vi "MonoSpec50 Find Ref Position_trig.vi"(2 "error in":errorcluster, 4 "Moving Ref":refnum<vi>) -> (0 "error out":errorcluster, 1 "Moving":bool caption="Déplacement\nen cours")   [LabVIEW 2012]
doc: "Ce VI envoie un train d'impulsion au moteur, pour le faire tourné dans la direction négative. Les impulsion sont générée en continu jusqu'à ce qu'un front montant soit détecté sur la ligne de détection de position de référence."
uses:
  <vilib>/Utility/error.llb/DialogType.ctl
  <vilib>/DAQmx/write.llb/DAQmx Write (Digital Bool 1Line 1Point).vi
  <vilib>/DAQmx/read.llb/DAQmx Read (Counter U32 1Chan 1Samp).vi
  <vilib>/DAQmx/miscellaneous.llb/DAQmx Fill In Error Info.vi
  <resource>/objmgr/daqmx.rc
panel:
  out "End":bool=TRUE
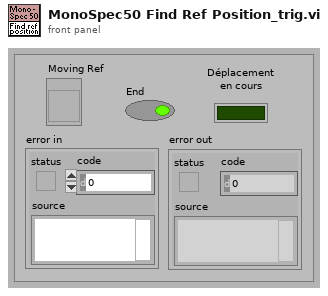
[diagram p1: front panel]
types:
  T1 = typedef "DialogType.ctl" = u16
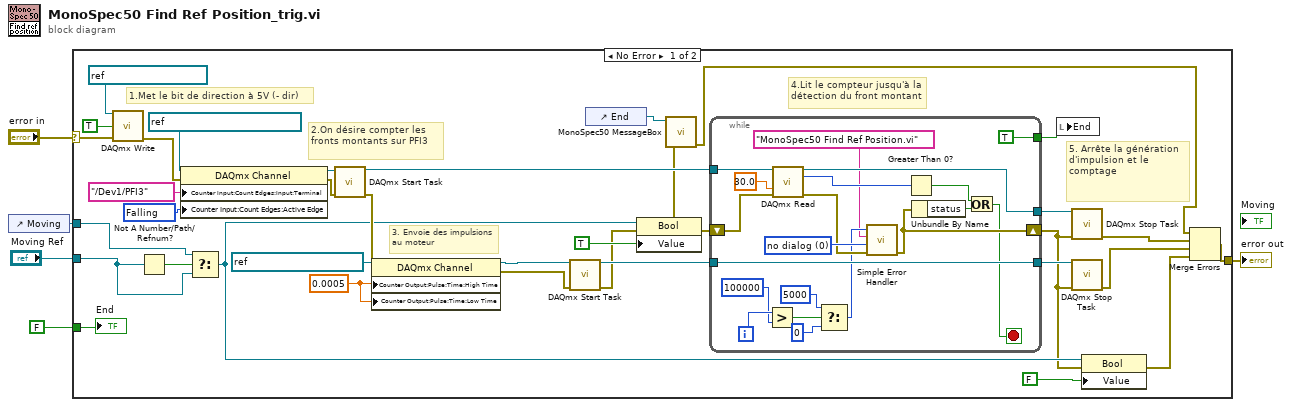
[diagram p0: block diagram]
diagram:
  n1 = control-ref of="Moving"() -> (w2:refnum<vi>)
  n2 = case shown="No Error" "error in" {
    selector: "error in" -> [w28 w61]
    tunnel: [w31 w61] -> w4
    tunnel: "Moving Ref" -> [w20 _]
    tunnel: w2 -> [w21 _]
    tunnel: FALSE ("End") -> [w12 _]
    frame No Error {
      w9 = 0.0005 ("CO.Pulse.HighTime")
      w29 = 10171 items=["Rising"=10280, "Falling"=10171] ("CI.CountEdges.ActiveEdge")
      # "5. Arrête la génération d'impulsion et le comptage"
      # "4.Lit le compteur jusqu'à la détection du front montant"
      # "3. Envoie des impulsions au moteur"
      # "2.On désire compter les fronts montants sur PFI3"
      # "1.Met le bit de direction à 5V (- dir)"
      n3 = call-poly <vilib>:"DAQmx Write.vi"("task/channels in"=refnum<k21> "Direction Spectro", "data"=TRUE, "error in"=w28) -> ("error out"=w25:errorcluster)  [unwired: 10 in, 2 out]
      n4 = Not A Number/Path/Refnum?(number/path/refnum=w20) -> (NaN/Path/Refnum?=w22:bool)
      n5 = property class="DAQmx Channel"(reference=refnum<k21> "ComptRefPulse Spectro" ("task"), error in=w25, "Counter Input:Count Edges:Input:Terminal"=tag "/Dev1/PFI3" ("CI.CountEdges.Term"), "Counter Input:Count Edges:Active Edge"=w29) -> (reference out=w37:refnum<k21>, error out=w36:errorcluster)
      n6 = Select(t=w21, s=w22, f=w20) -> (s? t:f=w17:refnum<vi>)
      n7 = call <vilib>:"DAQmx Start Task.vi"("task/channels in"=w37, "error in"=w36) -> ("task out"=w24:refnum<k21>, "error out"=w23:errorcluster)  [unwired: 12 in]
      n8 = property class="DAQmx Channel"(reference=refnum<k21> "Sortie Pulse Spectro" ("task/channels in"), error in=w23, "Counter Output:Pulse:Time:High Time"=w9, "Counter Output:Pulse:Time:Low Time"=w9) -> (reference out=w7:refnum<k21>, error out=w6:errorcluster)
      n9 = call <vilib>:"DAQmx Start Task.vi"("task/channels in"=w7, "error in"=w6) -> ("task out"=w35:refnum<k21>, "error out"=w18:errorcluster)  [unwired: 12 in]
      n10 = control-ref of="End"() -> (w13:refnum<vi>)
      n11 = property class="Bool"(reference=w17, error in=w18, "Value"=TRUE) -> (error out=w10:errorcluster)  [unwired: 1 out]
      n12 = call <userlib>:"MonoSpec50 MessageBox.vi"("error in (no error)"=w10, "End"=w13) -> ("error out"=w8:errorcluster)  [unwired: 5 in]
      n13 = while {
        tunnel: w24 -> [w60]
        tunnel: [w58] -> w39
        tunnel: w35 -> [w54]
        tunnel: [w54] -> w34
        shift-right: [w48] -> w16
        shift-left: w10 -> [w53]
        tunnel: [TRUE] -> w11
        i -> [w52]
        stop <- w43 stop-if-true
        w50 = T1 0 items=["no dialog", "OK message", "continue or stop message", "OK message + warnings", "continue/stop + warnings"] ("type of dialog (OK msg:1)")
        n14 = Greater?(x=w52, y=100000) -> (0:w47:bool)
        n15 = call-poly <vilib>:"DAQmx Read.vi"("task/channels in"=w60, "timeout"=30.0, "error in"=w53) -> ("task out"=w58:refnum<k21>, "data"=w59:u32, "error out"=w49:errorcluster)  [unwired: 10 in]
        n16 = Select(t=5000 ("error code (no error:0)"), s=w47, f=0) -> (s? t:f=w44:i32)
        n17 = call <vilib>:"Simple Error Handler.vi"("error code (no error:0)"=w44, "error source (\" \")"="MonoSpec50 Find Ref Position.vi" ("error source (\" \")"), "type of dialog (OK msg:1)"=w50, "error in (no error)"=w49) -> ("error out"=w48:errorcluster)  [unwired: 1 in, 4 out]
        n18 = Greater Than 0?(x=w59) -> (x > 0?=w55:bool)
        n19 = Unbundle By Name(w48) -> ("status"=w56:bool)
        n20 = Or(x=w55, y=w56) -> (x .or. y?=w43:bool)
      }
      n21 = local write "End"(w11) -> ()
      n22 = call <vilib>:"DAQmx Stop Task.vi"("task/channels in"=w39, "error in"=w16) -> ("error out"=w33:errorcluster)  [unwired: 12 in, 1 out]
      n23 = call <vilib>:"DAQmx Stop Task.vi"("task/channels in"=w34, "error in"=w16) -> ("error out"=w32:errorcluster)  [unwired: 12 in, 1 out]
      n24 = property class="Bool"(reference=w17, error in=w16, "Value"=FALSE) -> (error out=w15:errorcluster)  [unwired: 1 out]
      n25 = Merge Errors(w8, w33, w32, w15) -> (w31:errorcluster)
      "End" <- w12
    }
    frame Error {
    }
  }
  "error out" <- w4
